vi "Check_3_Subsequent_Problem_Points_Subtrack-1.vi"(1 "[IN] Subtracks":T1(array[cluster])) -> (0 "[OUT] 3 Subsequent problem points in subtrack":bool)   [LabVIEW 2013]
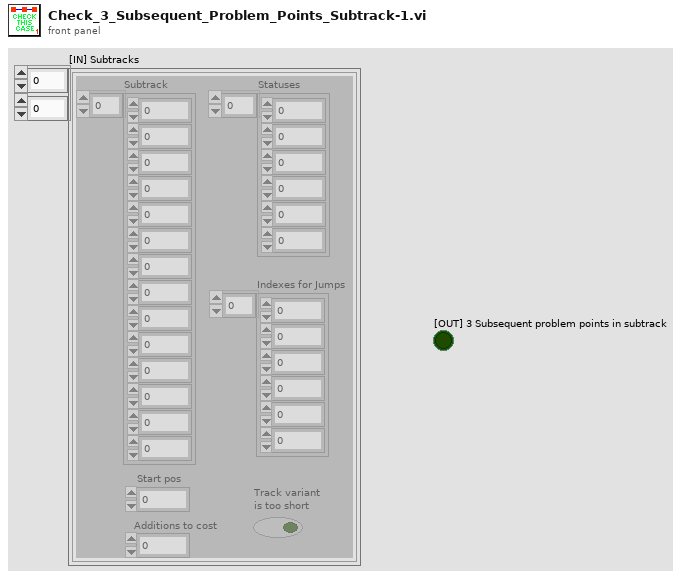
[diagram p1: front panel]
types:
  T1 = cluster{"Subtrack":dbl[], "Statuses":i16[], "Start pos":i32, "Additions to cost":i32, "Track variant \nis too short":bool, "Indexes for Jumps":i32[]}[][]
  T2 = cluster{"Subtrack":dbl[], "Statuses":i16[], "Start pos":i32, "Additions to cost":i32, "Track variant \nis too short":bool, "Indexes for Jumps":i32[]}[]
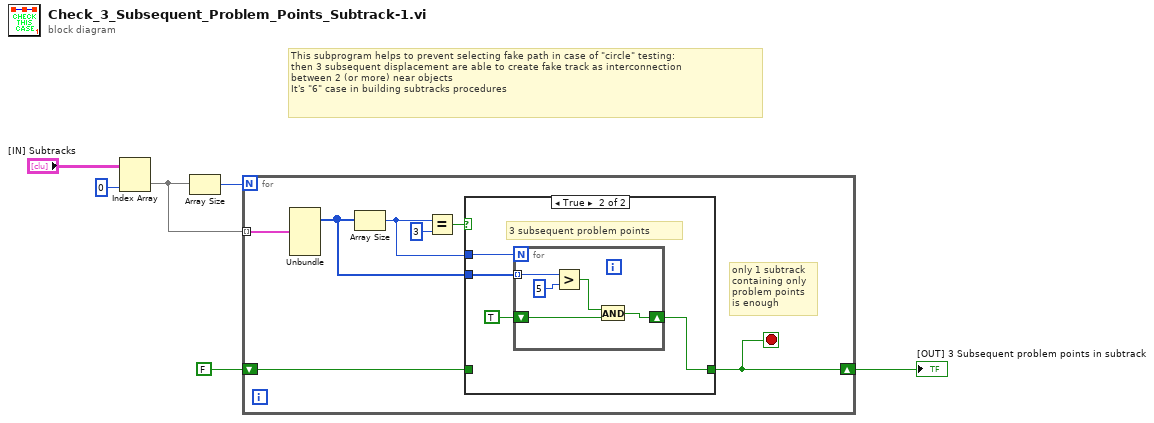
[diagram p0: block diagram]
diagram:
  # "This subprogram helps to prevent selecting fake path in case of \"circle\" testing:\nthen 3 subsequent displacement are able to create fake track as interconnection \nbetween 2 (or more) near objects\nIt's \"6\" case in building subtracks procedures"
  n1 = Index Array(array="[IN] Subtracks", index (col)=0 ("disabled index (col)")) -> (element=w3:T2)  [unwired: 1 in]
  n2 = Array Size(array=w3) -> (size(s)=w4:i32)
  n3 = for {
    N: w4 -> [_]
    tunnel: w3 -> [w13] mode=indexing
    shift-right: [w7] -> w1
    shift-left: FALSE -> [w8]
    stop <- w7 stop-if-true
    # "only 1 subtrack \ncontaining only \nproblem points \nis enough"
    n4 = Unbundle(w13) -> ("Statuses"=w9:i16[])  [unwired: 5 out]
    n5 = Array Size(array=w9) -> (size(s)=w10:i32)
    n6 = Equal?(x=w10, y=3) -> (x = y?=w11:bool)
    n7 = case shown="True" w11 {
      tunnel: w10 -> [_ w18]
      tunnel: w9 -> [_ w17]
      tunnel: w8 -> [w14 _]
      tunnel: [w14 w15] -> w7
      frame False {
        # "other type of subtrack\n(maybe too short, maybe\ntoo long)"
      }
      frame True {
        # "3 subsequent problem points"
        n8 = for {
          N: w18 -> [_]
          tunnel: w17 -> [w23] mode=indexing
          shift-right: [w20] -> w15
          shift-left: TRUE -> [w21]
          n9 = Greater?(x=w23, y=i16 5 ("element")) -> (0:w19:bool)
          n10 = And(x=w19, y=w21) -> (x .and. y?=w20:bool)
        }
      }
    }
  }
  "[OUT] 3 Subsequent problem points in subtrack" <- w1
